vi "Process Mouse Move.vi"(0 "Listbox":refnum<vi>, 1 "Color Box":refnum<vi>, 5 "State in":T1, 7 "Coords":T6, 11 "error in (no error)":errorcluster) -> (6 "State out":T1, 15 "error out":errorcluster)   [LabVIEW 2020, in "KTable.xctl"]
uses:
  KTable.xctl
  <vilib>/Utility/miscctls.llb/LVPoint32TypeDef.ctl
  State.ctl
  ColumnSpec.ctl
  ColumnType.ctl
  Table Properties.ctl
  Events.ctl
  Event Data.ctl
  Event Type.ctl
  <vilib>/Utility/miscctls.llb/LVPositionTypeDef.ctl
  Array Manipulation VIs/Array-Dimensions (2D string).vi
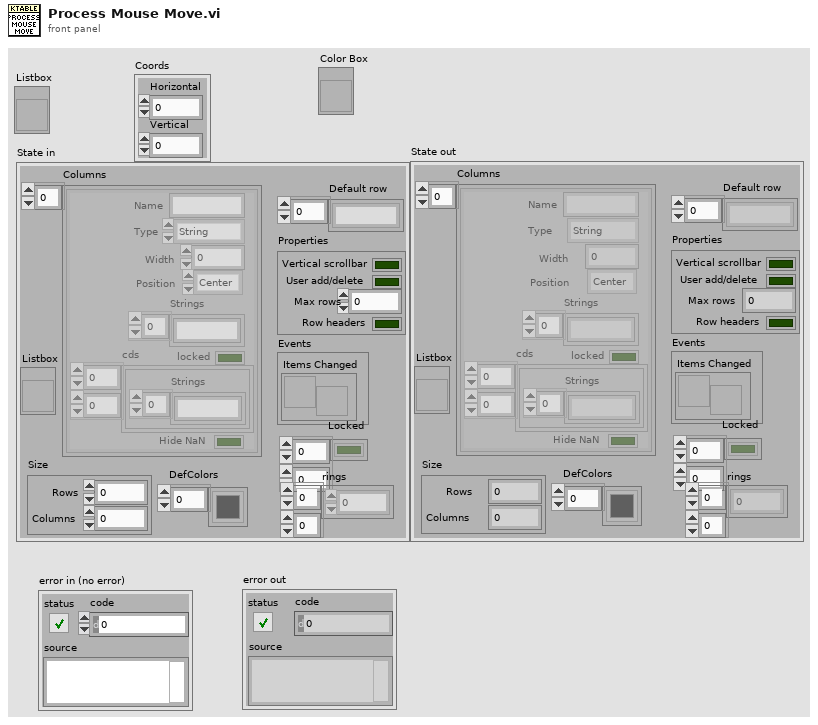
[diagram p1: front panel]
types:
  T1 = typedef "KTable.xctl/State.ctl" = cluster{"Columns":T2[], "Listbox":refnum<vi>, "Default row":string[], "Properties":T4, "Events":T5, "Locked":bool[][], "Size":cluster{"Rows":i32, "Columns":i32}, "rings":i32[][], "DefColors":u32[]}
  T2 = typedef "KTable.xctl/ColumnSpec.ctl" = cluster{"Name":string, "Type":T3, "Width":i32, "Strings":string[], "Position":enum16{"Left", "Center", "Right"}, "locked":bool, "cds":cluster{"Strings":string[]}[][], "Hide NaN":bool}
  T3 = typedef "KTable.xctl/ColumnType.ctl" = enum16{"String", "Enum", "Int", "Double", "Boolean", "Ring", "Formula", "Color"}
  T4 = typedef "KTable.xctl/Table Properties.ctl" = cluster{"Vertical scrollbar":bool, "User add/delete":bool, "Max rows":i32, "Row headers":bool}
  T5 = typedef "KTable.xctl/Events.ctl" = cluster{"Items Changed":refnum<user-event>}
  T6 = typedef "LVPoint32TypeDef.ctl" = cluster{"Horizontal":i32, "Vertical":i32}
  T7 = typedef "LVRowAndColumnTypeDef.ctl" = cluster{"Row":i32, "Column":i32}
  T8 = typedef "LVPositionTypeDef.ctl" = cluster{"Left":i32, "Top":i32}
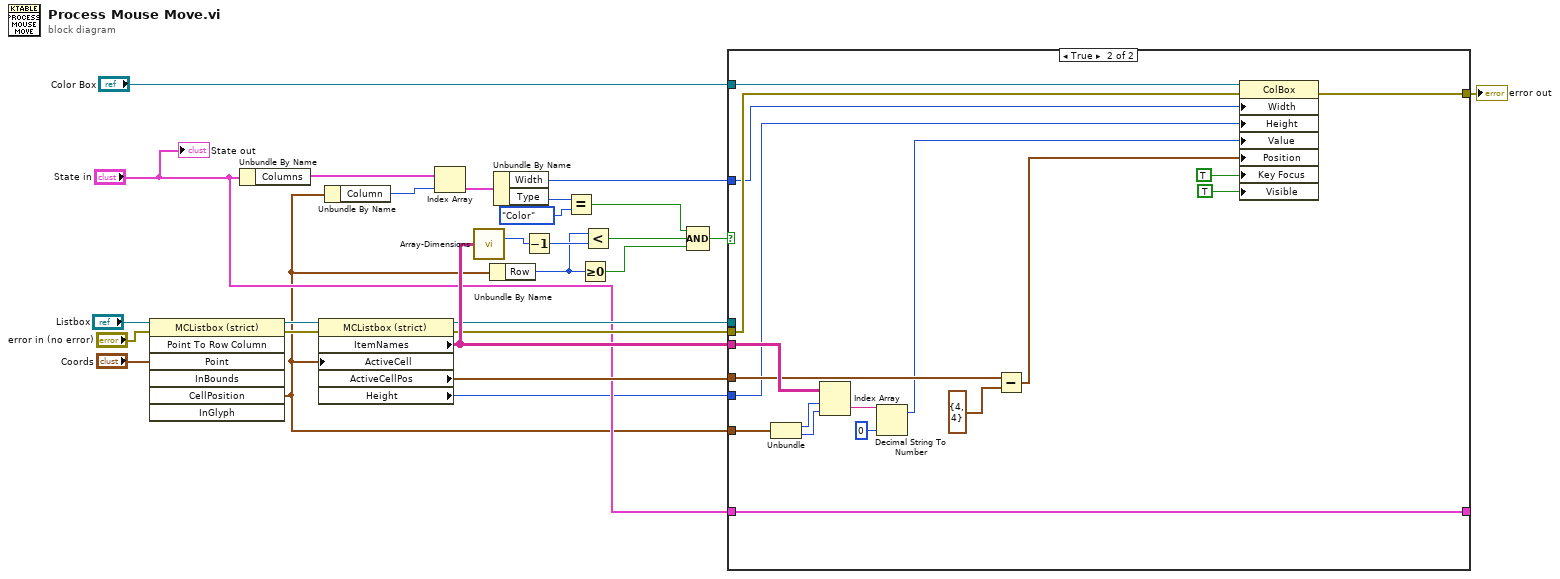
[diagram p0: block diagram]
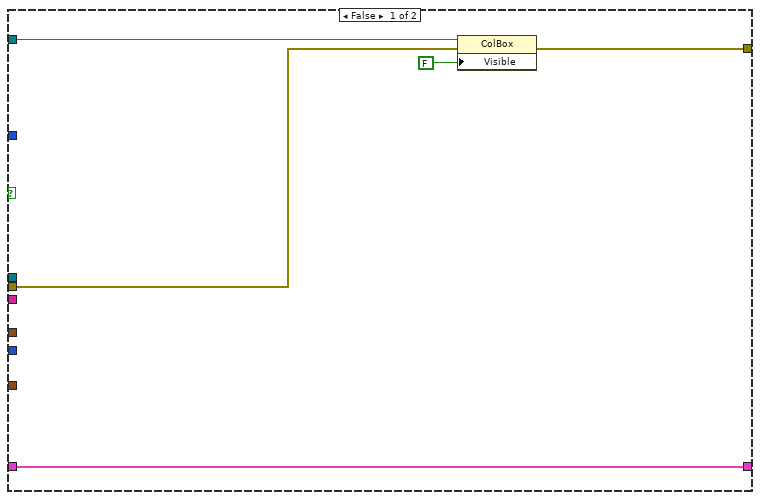
[diagram p2: hidden frame]
diagram:
  n1 = invoke on="Invoke Node" class="MCListbox (strict)" method="Point To Row Column"(reference="Listbox", error in="error in (no error)", "Point"="Coords") -> (reference out=w23:refnum<vi>, error out=w22:errorcluster, "CellPosition"=w10:T7)  [unwired: 4 in, 4 out]
  n2 = Unbundle By Name("State in") -> ("Columns"=w16:T2[])
  n3 = property class="MCListbox (strict)"(reference=w23, error in=w22, "ActiveCell"=w10) -> (reference out=w14:refnum<vi>, error out=w19:errorcluster, "ItemNames"=w20:string[][], "ActiveCellPos"=w21:T8, "Height"=w1:u32)
  n4 = Unbundle By Name(w10) -> ("Column"=w15:i32)
  n5 = Index Array(array=w16, index=w15) -> (element=w25:T2)
  n6 = call-poly "Array-Dimensions.vi"("2D Array"=w20) -> ("# rows"=w9:i32)  [unwired: 13 in, 1 out]
  n7 = Unbundle By Name(w10) -> ("Row"=w8:i32)
  n8 = Unbundle By Name(w25) -> ("Width"=w17:i32, "Type"=w4:T3)
  n9 = Decrement(x=w9) -> (x-1=w11:i32)
  n10 = Equal?(x=w4, y=ColumnType."Color") -> (x = y?=w2:bool)
  n11 = Greater Or Equal To 0?(x=w8) -> (x >= 0?=w6:bool)
  n12 = Less?(x=w8, y=w11) -> (x < y?=w7:bool)
  n13 = Compound Arithmetic op=AND(w2, w7, w6) -> (w5:bool)
  n14 = case shown="True" w5 {
    tunnel: "Color Box" -> [w31 w48]
    tunnel: w21 -> [_ w38]
    tunnel: w20 -> [_ w44]
    tunnel: w19 -> [w30 w47]
    tunnel: [w29 w46] -> w18
    tunnel: w17 -> [_ w40]
    tunnel: w10 -> [_ w45]
    tunnel: w14 -> [_ _]
    tunnel: "State in" -> [w28 w41]
    tunnel: [w28 w41] -> _
    tunnel: w1 -> [_ w36]
    frame False {
      n15 = property on="Property Node" class="ColBox"(reference=w31, error in=w30, "Visible"=FALSE) -> (error out=w29:errorcluster)  [unwired: 1 out]
    }
    frame True {
      n16 = Unbundle(w45) -> ("Row"=w42:i32, "Column"=w43:i32)
      n17 = Index Array(array=w44, index (row)=w42, index (col)=w43) -> (element=w35:string)
      n18 = Decimal String To Number(string=w35, default (0L)=u32 0 ("default (0 I32)")) -> (offset past number=w33:i32)  [unwired: 1 in, 1 out]
      n19 = Subtract(x=w38, y=T8 {"Left"=4, "Top"=4}) -> (x-y=w39:T8)
      n20 = property on="Property Node" class="ColBox"(reference=w48, error in=w47, "Width"=w40, "Height"=w36, "Value"=w33, "Position"=w39, "Key Focus"=TRUE, "Visible"=TRUE) -> (error out=w46:errorcluster)  [unwired: 1 out]
    }
  }
  "error out" <- w18
  "State out" <- "State in"
